vi "Get Fit Cursor Position.vi"(0 "Graph Reference":refnum<vi>) -> (1 "Force (pN)":dbl, 2 "Extension (nm)":dbl)   [LabVIEW 2013]
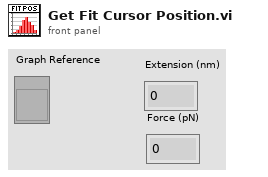
[diagram p1: front panel]
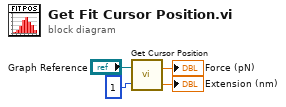
[diagram p0: block diagram]
diagram:
  n1 = call "Get Cursor Position.vi"("Cursor ID"=u32 1 ("Active Cursor"), "Graph Reference"="Graph Reference") -> ("X Position"=→"Extension (nm)":dbl, "Y Position"=→"Force (pN)":dbl)
